vi "holoComp1.vi"(7 "Beam Parameters, dependant on SLM and LASER  B":T2={"amplitude matrix"=[], "number of columns in amplitude matrix"=1400, "number of rows in amplitude matrix"=1050, "represented width (in m)"=0.01498, "represented height (in m)"=0.01092, "wavelength (in m)"=6.33e-07}, 8 "No.of Quadrants 2":i32=6 min=0 max=90, 9 "Pie Cut Phase (Degrees) 2":T1 {"1" min=0.0 max=360.0 step=180.0; "2" min=0.0 max=360.0 step=180.0; "3" min=0.0 max=360.0 step=180.0; "4" min=0.0 max=360.0 step=180.0; "5" min=0.0 max=360.0 step=180.0; "6" min=0.0 max=360.0 step=180.0}, 10 "Pie cut separation (degrees) 2":i32=5 max=90, 11 "thetaIn":sgl[][](array[numeric])) -> (2 "thetaOut":dbl[][](array[numeric]), 3 "Pie Cut Phase 2":dbl[][](graph))   [LabVIEW 2020]
uses:
  <vilib>/express/express arith-compare/Formula/XNode/ExpressFormulaBlockNode.xnode
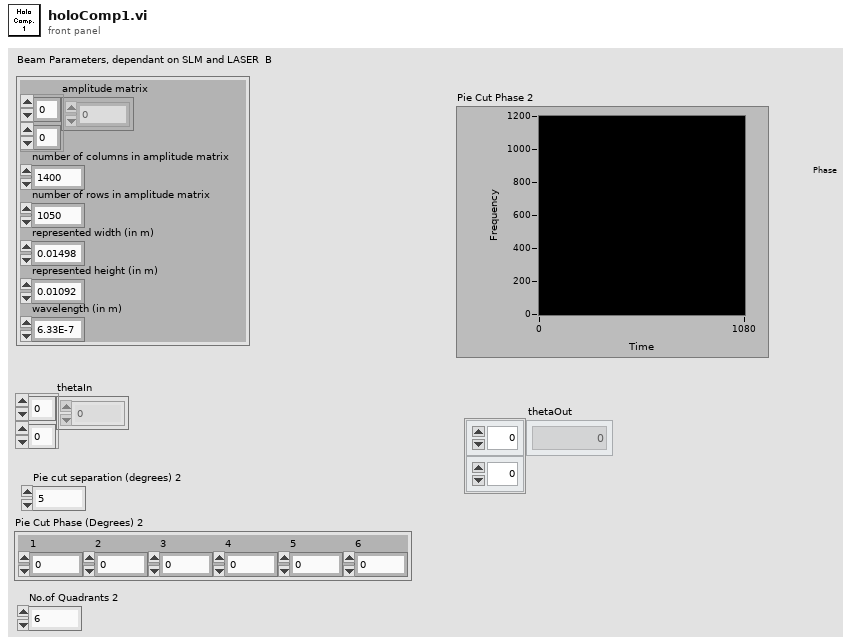
[diagram p1: front panel]
types:
  T1 = cluster{"1":dbl, "2":dbl, "3":dbl, "4":dbl, "5":dbl, "6":dbl}
  T2 = cluster{"amplitude matrix":csg[][], "number of columns in amplitude matrix":i32, "number of rows in amplitude matrix":i32, "represented width (in m)":dbl, "represented height (in m)":dbl, "wavelength (in m)":dbl}
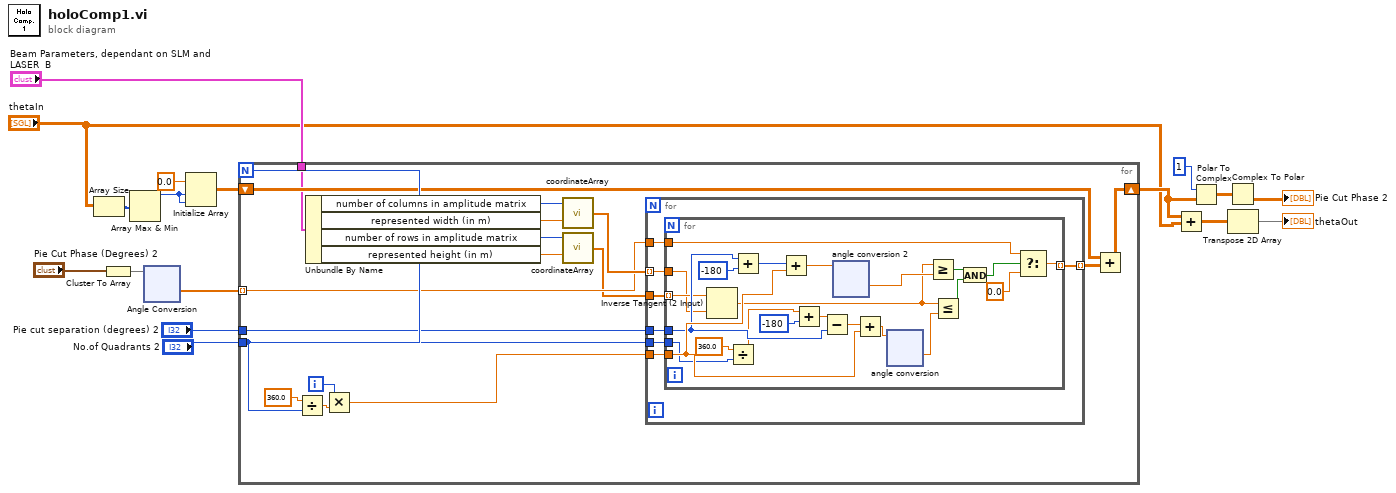
[diagram p0: block diagram]
diagram:
  n1 = Array Size(array="thetaIn") -> (size(s)=w15:i32[])
  n2 = Cluster To Array(cluster="Pie Cut Phase (Degrees) 2") -> (array=w13:dbl[])
  n3 = Array Max & Min(array=w15) -> (max value=w14:i32)  [unwired: 3 out]
  n4 = xnode ("Angle Conversion")("X"=w13) -> ("Result"=w12:dbl[])  [unwired: 1 in, 1 out]
  n5 = Initialize Array(0.0 ("element"), w14, w14) -> (w17:dbl[][])
  n6 = for {
    N: "No.of Quadrants 2" -> [_]
    shift-right: [w27] -> w10
    shift-left: w17 -> [w28]
    tunnel: "Pie cut separation (degrees) 2" -> [w26]
    tunnel: "No.of Quadrants 2" -> [w20]
    tunnel: w12 -> [w23] mode=indexing
    tunnel: "Beam Parameters, dependant on SLM and LASER  B" -> [w19]
    i -> [w22]
    n7 = Divide(x=360.0, y=w20) -> (x/y=w24:dbl)
    n8 = Unbundle By Name(w19) -> ("number of columns in amplitude matrix"=w34:i32, "represented width (in m)"=w33:dbl, "number of rows in amplitude matrix"=w32:i32, "represented height (in m)"=w31:dbl)
    n9 = Multiply(x=w22, y=w24) -> (x*y=w29:dbl)
    n10 = call "coordinateArray.vi"("width of represented x (or y) range (in m; default 1E-3=1mm)"=w33, "array size (default 64)"=w34) -> ("x array"=w30:sgl[])
    n11 = call "coordinateArray.vi"("width of represented x (or y) range (in m; default 1E-3=1mm)"=w31, "array size (default 64)"=w32) -> ("x array"=w18:sgl[])
    n12 = for {
      tunnel: w18 -> [w41]
      tunnel: w30 -> [w40] mode=indexing
      tunnel: [w39] -> w21 mode=indexing
      tunnel: w29 -> [w38]
      tunnel: w26 -> [w37]
      tunnel: w20 -> [w36]
      tunnel: w23 -> [w35]
      n13 = for {
        tunnel: w41 -> [w47] mode=indexing
        tunnel: w40 -> [w46]
        tunnel: [w44] -> w39 mode=indexing
        tunnel: w38 -> [w58]
        tunnel: w37 -> [w54]
        tunnel: w36 -> [w52]
        tunnel: w35 -> [w45]
        n14 = Inverse Tangent (2 Input)(1:w46, 2:w47) -> (0:w43:sgl)
        n15 = Divide(x=360.0, y=w52) -> (x/y=w50:dbl)
        n16 = Add(x=w54, y=-180) -> (x+y=w56:i32)
        n17 = Add(x=w56, y=w58) -> (x+y=w59:dbl)
        n18 = Add(x=w50, y=-180) -> (x+y=w48:dbl)
        n19 = Subtract(x=w48, y=w54) -> (x-y=w55:dbl)
        n20 = xnode ("angle conversion 2")("X1"=w59) -> ("Result"=w60:dbl)  [unwired: 1 in, 1 out]
        n21 = Add(x=w55, y=w58) -> (x+y=w57:dbl)
        n22 = xnode ("angle conversion")("X1"=w57) -> ("Result"=w42:dbl)  [unwired: 1 in, 1 out]
        n23 = Greater Or Equal?(x=w43, y=w60) -> (x >= y?=w64:bool)
        n24 = Less Or Equal?(x=w43, y=w42) -> (x <= y?=w63:bool)
        n25 = And(x=w64, y=w63) -> (x .and. y?=w62:bool)
        n26 = Select(t=w45, s=w62, f=0.0) -> (s? t:f=w44:dbl)
      }
    }
    n27 = Add(x=w28, y=w21) -> (x+y=w27:dbl[][])
  }
  n28 = Add(x=w10, y="thetaIn") -> (x+y=w11:dbl[][])
  n29 = Polar To Complex(1:w10, 2:1) -> (0:w8:cdb[][])
  n30 = Complex To Polar(r * e^(i*theta)=w8) -> (theta=→"Pie Cut Phase 2":dbl[][])  [unwired: 1 out]
  n31 = Transpose 2D Array(2D array=w11) -> (transposed array=→"thetaOut":dbl[][])
